vi "pipx40 VXIPnp Error Converter.vi"(2 "error in (no error)":errorcluster {"code" format="%.0x"}, 3 "name of VI (\"\")":string, 4 "VXIPnp error code (0)":i32, 5 "instrument handle":i32) -> (0 "error out":errorcluster {"code" format="%.0x"}, 1 "instrument handle out":i32)   [LabVIEW 2011]
doc: "This VI converts error codes from VXIPnp instrument driver to standard LabVIEW error codes. If an error is detected the VI builds the appropriate error cluster that is readable by one of the error handlers supplied with LabVIEW."
uses:
  pipx40_32.dll
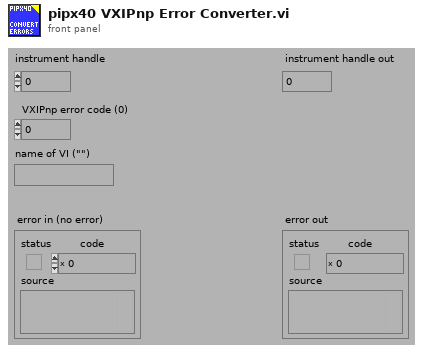
[diagram p1: front panel]
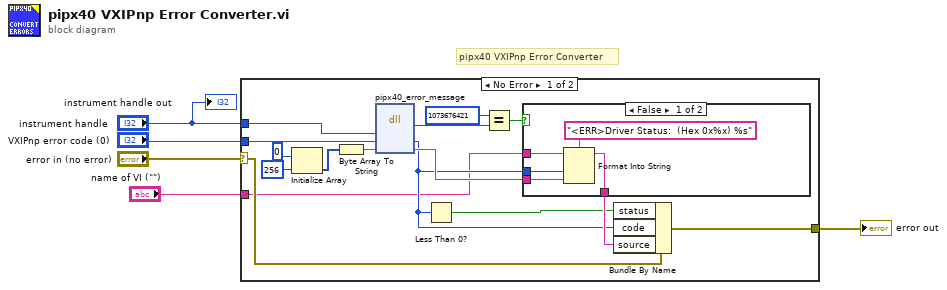
[diagram p0: block diagram]
diagram:
  # "pipx40 VXIPnp Error Converter"
  n1 = case shown="No Error" "error in (no error)" {
    selector: "error in (no error)" -> [w7 w28]
    tunnel: "VXIPnp error code (0)" -> [w21 _]
    tunnel: [w20 w28] -> w2
    tunnel: "instrument handle" -> [w15 _]
    tunnel: "name of VI (\"\")" -> [w6 _]
    frame No Error {
      n2 = Initialize Array(u8 0, 256) -> (w18:u8[])
      n3 = Byte Array To String(unsigned byte array=w18) -> (string=w16:string)
      n4 = dll-call lib="pipx40_32.dll" fn="pipx40_error_message" label="pipx40 VXIPnp Error Converter"(w15, w21, w16) -> (w13:i32, w8:i32, w11:string)  [unwired: 4 in, 2 out]
      n5 = Less Than 0?(x=w8) -> (x < 0?=w9:bool)
      n6 = Equal?(x=1073676421 ("y"), y=w13) -> (x = y?=w12:bool)
      n7 = case shown="False" w12 {
        tunnel: w11 -> [w24 _]
        tunnel: w6 -> [w26 w27]
        tunnel: w8 -> [w25 _]
        tunnel: [w23 w27] -> w10
        frame False {
          n8 = Format Into String(format string="<ERR>Driver Status:  (Hex 0x%x) %s", initial string=w26, w25, w24) -> (resulting string=w23:string)  [unwired: 1 in, 1 out]
        }
        frame True {
        }
      }
      n9 = Bundle By Name(cluster=w7, "status"=w9, "code"=w8, "source"=w10) -> (w20:errorcluster)
    }
    frame Error {
    }
  }
  "error out" <- w2
  "instrument handle out" <- "instrument handle"
